vi "Sets the GB HI SET resistance value for MANU.vi"(5 "Enable to Query":bool, 7 "Enable to Setup":bool, 8 "error in":errorcluster, 10 "GB HI SET resistance value(m£[)":sgl=650.0 min=0.1 max=650 format="%.1f", 11 "VISA resource name":refnum<visa-resource-name>) -> (0 "error out":errorcluster, 2 "Return the GB HI SET resistance value":string, 3 "VISA resource name out":refnum<visa-resource-name>)   [LabVIEW 2011, in "GPT-9000.lvlib"]
uses:
  <instrlib>/GPT-9000/GPT-9000.lvlib
panel:
  # "m£["
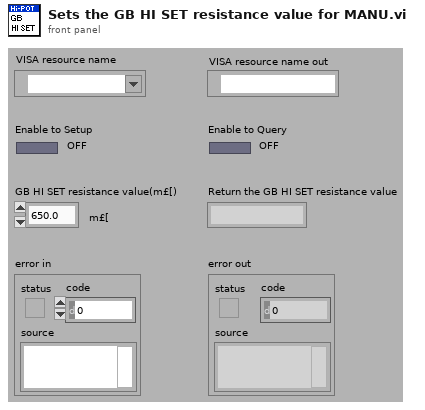
[diagram p1: front panel]
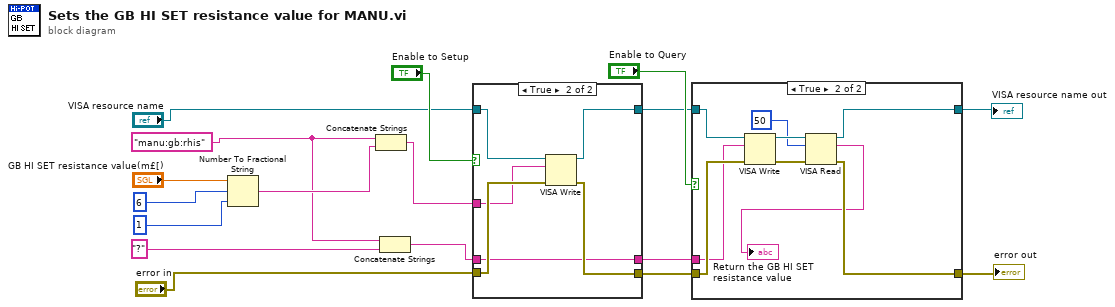
[diagram p0: block diagram]
diagram:
  w12 = "manu:gb:rhis"
  n1 = Number To Fractional String(number="GB HI SET resistance value(m£[)", width (-)=i16 6, precision (6)=i16 1) -> (F-format string=w14:string)  [unwired: 1 in]
  n2 = Concatenate Strings(w12, w14) -> (w10:string)
  n3 = Concatenate Strings(w12, "?") -> (w9:string)
  n4 = case shown="True" "Enable to Setup" {
    tunnel: w10 -> [_ w24]
    tunnel: w9 -> [w18 w21]
    tunnel: "VISA resource name" -> [w19 w26]
    tunnel: "error in" -> [w20 w25]
    tunnel: [w20 w22] -> w4
    tunnel: [w19 w23] -> w5
    tunnel: [w18 w21] -> w3
    frame False {
    }
    frame True {
      n5 = VISA Write(VISA resource name=w26, write buffer=w24, error in (no error)=w25) -> (VISA resource name out=w23:refnum<visa-resource-name>, error out=w22:errorcluster)  [unwired: 1 out]
    }
  }
  n6 = case shown="True" "Enable to Query" {
    tunnel: w5 -> [w28 w34]
    tunnel: w4 -> [w27 w33]
    tunnel: w3 -> [_ w32]
    tunnel: [w28 w31] -> w2
    tunnel: [w27 w30] -> w1
    frame False {
    }
    frame True {
      n7 = VISA Write(VISA resource name=w34, write buffer=w32, error in (no error)=w33) -> (VISA resource name out=w36:refnum<visa-resource-name>, error out=w37:errorcluster)  [unwired: 1 out]
      n8 = VISA Read(VISA resource name=w36, byte count=u32 50, error in (no error)=w37) -> (VISA resource name out=w31:refnum<visa-resource-name>, read buffer=→"Return the GB HI SET resistance value":string, error out=w30:errorcluster)  [unwired: 1 out]
    }
  }
  "VISA resource name out" <- w2
  "error out" <- w1
